vi "Increment Run Count.vi"(8 "error in (no error)":errorcluster, 11 "Result Table.lvclass":refnum<class "Result Table.lvclass">) -> (0 "error out":errorcluster, 3 "Result Table":refnum<class "Result Table.lvclass">)   [LabVIEW 2020, in "Result Table.lvclass"]
uses:
  Result Table.lvclass
  Result Table.lvclass/Result Table.ctl
  TypeDefs/Table Columns.ctl
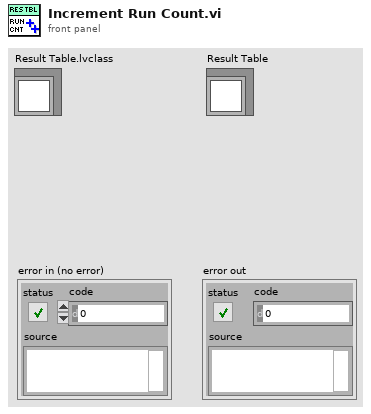
[diagram p1: front panel]
types:
  T1 = typedef "Result Table.lvclass/Table Columns.ctl" = u16
  T2 = typedef "Results.ctl" = cluster{"Method Count":u32, "Executed Methods":u32, "Passed Methods":u32, "Failed Methods":u32, "Method Errors":u32, "Skipped Method":u32}
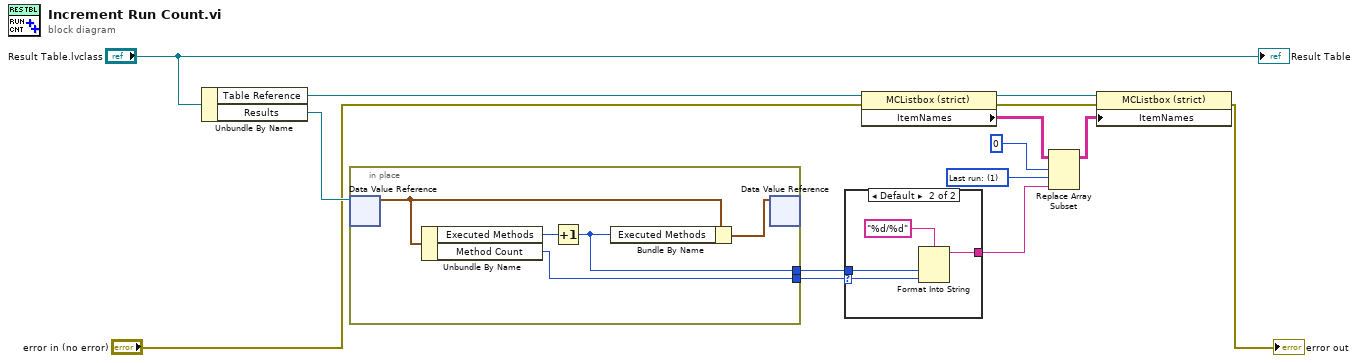
[diagram p0: block diagram]
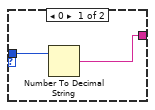
[diagram p2: hidden frame]
diagram:
  w11 = T1 1 items=["Last run:"=1, "Passed:"=3, "Failed:"=5, "Errors:"=7, "Skipped"=9] ("Table Columns")
  n1 = Unbundle By Name("Result Table.lvclass") -> ("Table Reference"=w6:refnum<vi>, "Results"=w13:refnum<data-value>)
  n2 = in-place {
    in-place-border: [w16] -> w2
    in-place-border: [w15] -> w1
    n3 = in-place-dvr #1(w13) -> (w18:T2)  [unwired: 1 out]
    n4 = Unbundle By Name(w18) -> ("Executed Methods"=w17:u32, "Method Count"=w15:u32)
    n5 = Increment(x=w17) -> (x+1=w16:u32)
    n6 = Bundle By Name(cluster=w18, "Executed Methods"=w16) -> (w19:T2)
    n7 = in-place-dvr #1(w19) -> ()  [unwired: 2 out]
  }
  n8 = case shown="Default" w1 {
    selector: w1 -> [_ w22]
    tunnel: [w20 w24] -> w3
    tunnel: w2 -> [w21 w23]
    frame 0 {
      n9 = Number To Decimal String(number=w21) -> (decimal integer string=w20:string)  [unwired: 1 in]
    }
    frame Default {
      n10 = Format Into String(format string="%d/%d", w23, w22) -> (resulting string=w24:string)  [unwired: 2 in, 1 out]
    }
  }
  n11 = property class="MCListbox (strict)"(reference=w6, error in="error in (no error)") -> (reference out=w7:refnum<vi>, error out=w8:errorcluster, "ItemNames"=w12:string[][])
  n12 = Replace Array Subset(array=w12, new element=w3, index (row)=0 ("disabled index (row)"), index (col)=w11) -> (w9:string[][])
  n13 = property class="MCListbox (strict)"(reference=w7, error in=w8, "ItemNames"=w9) -> (error out=→"error out":errorcluster)  [unwired: 1 out]
  "Result Table" <- "Result Table.lvclass"
